vi "Cfg List _ Index Col PopUp Types.vi"(8 "error in":errorcluster caption="错误输入", 10 "ColHeaders[]":string[](array[string]), 11 "Chan Para":T3) -> (0 "error out":errorcluster caption="错误输出", 2 "ColPopupTypes[]":T1[](array[typedef]))   [LabVIEW 2016]
uses:
  HardWare/Ctrls/HardWare _ Channel Configurations PopUp Type.ctl
  ToolKit/Popup/Private/Ctrls/POP_Data Type.ctl
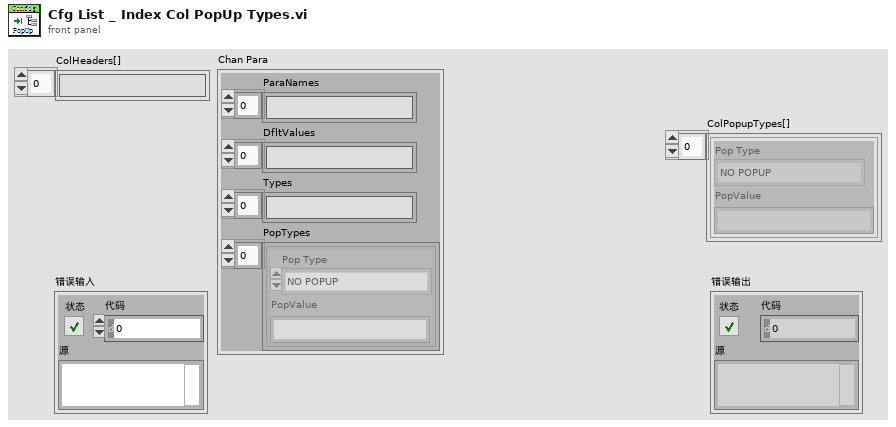
[diagram p1: front panel]
types:
  T1 = typedef "HardWare _ Channel Configurations PopUp Type.ctl" = cluster{"Pop Type":T2, "PopValue":string}
  T2 = typedef "POP_Data Type.ctl" = enum16{"NO POPUP", "Unkown", "String", "Integer", "Float", "Color", "Boolean", "Ring", "Captioned String", "Captioned Integer", "Button Color", "2 Int Cluster", "4 Int Cluster", "6-Dbl Cluster", "Path", "Combox", "Time", "ShotCut String"}
  T3 = cluster{"ParaNames":string[], "DfltValues":string[], "Types":string[], "PopTypes":T1[]}
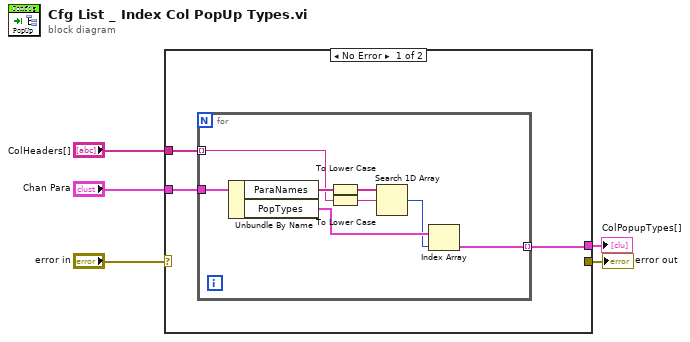
[diagram p0: block diagram]
diagram:
  n1 = case shown="No Error" "error in" {
    selector: "error in" -> [_ w17]
    tunnel: [_ w17] -> w4
    tunnel: "ColHeaders[]" -> [w8 _]
    tunnel: "Chan Para" -> [w7 _]
    tunnel: [w6 _] -> w1
    frame No Error {
      n2 = for {
        tunnel: w8 -> [w14] mode=indexing
        tunnel: w7 -> [w16]
        tunnel: [w11] -> w6 mode=indexing
        n3 = Unbundle By Name(w16) -> ("ParaNames"=w15:string[], "PopTypes"=w13:T1[])
        n4 = To Lower Case(string=w15) -> (all lower case string=w10:string[])
        n5 = To Lower Case(string=w14) -> (all lower case string=w9:string)
        n6 = Search 1D Array(1D array=w10, element=w9) -> (index of element=w12:i32)  [unwired: 1 in]
        n7 = Index Array(array=w13, index=w12) -> (element=w11:T1)
      }
    }
    frame Error {
    }
  }
  "error out" <- w4
  "ColPopupTypes[]" <- w1
